vi "Folder Names.vi"() -> ()   [LabVIEW 2016]
panel:
  out "Log Path":path
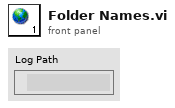
[diagram p1: front panel]
diagram:
